vi "HW_Gantner_Get Save T0.vi"(5 "dt":dbl format="%#_13g", 7 "data length":i32, 9 "error in":errorcluster, 10 "StartT0":timestamp, 11 "T0 in":timestamp) -> (1 "error out":errorcluster, 2 "TimeCh data":waveform(dbl), 3 "T0 out":timestamp)   [LabVIEW 2016]
uses:
  Ctrls/Continuous Operations.ctl
  Ctrls/GlobeVaribles.vi
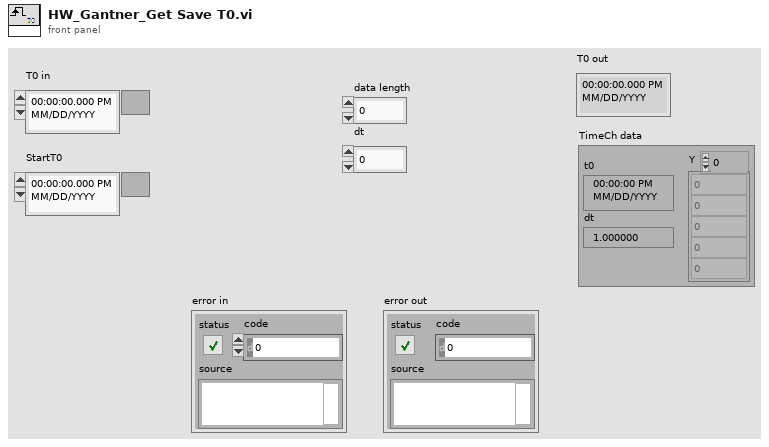
[diagram p1: front panel]
types:
  T1 = typedef "Continuous Operations.ctl" = enum16{"Writting", "Pause", "Stop"}
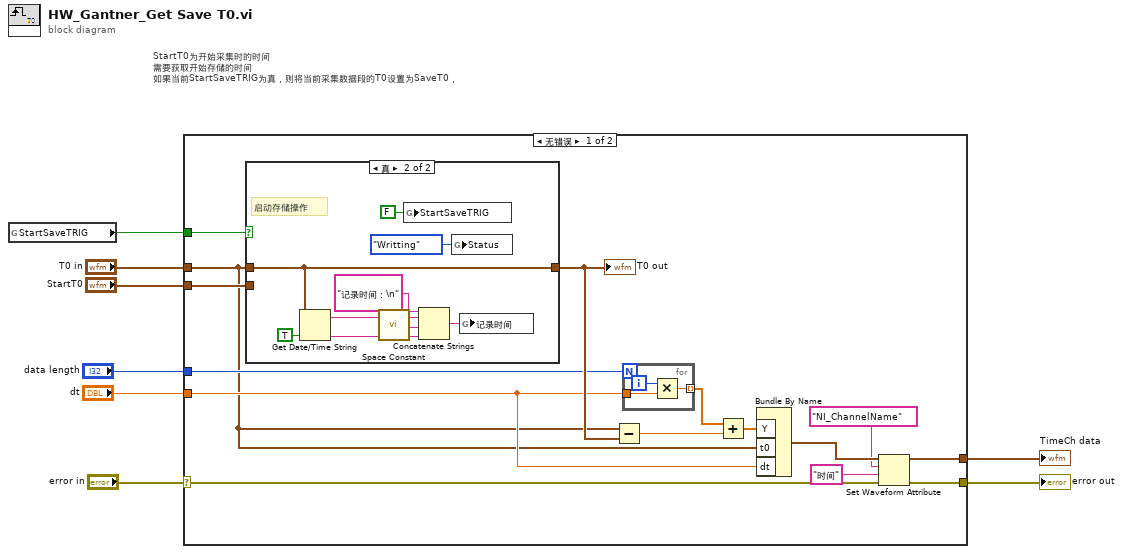
[diagram p0: block diagram]
diagram:
  # "StartT0为开始采集时的时间\n需要获取开始存储的时间\n如果当前StartSaveTRIG为真，则将当前采集数据段的T0设置为SaveT0，"
  n1 = global read "GlobeVaribles.vi" "StartSaveTRIG"() -> (w7:bool)
  n2 = case shown="无错误" "error in" {
    selector: "error in" -> [w12 w37]
    tunnel: "StartT0" -> [w23 _]
    tunnel: w7 -> [w22 _]
    tunnel: "T0 in" -> [w10 _]
    tunnel: "data length" -> [w14 _]
    tunnel: "dt" -> [w13 _]
    tunnel: [w11 w37] -> w2
    tunnel: [w9 _] -> w1
    frame No Error {
      n3 = case shown="真" w22 {
        tunnel: w10 -> [_ w34]
        tunnel: [w27 w34] -> w15
        tunnel: w23 -> [w27 _]
        frame False {
        }
        frame True {
          # "启动存储操作"
          n4 = Get Date/Time String(seconds (now)=w34, want seconds? (F)=TRUE ("需要秒？(F)")) -> (date string=w33:string, time string=w32:string)  [unwired: 1 in]
          n5 = call <vilib>:"Space Constant.vi"() -> ("String"=w29:string)
          n6 = global write "GlobeVaribles.vi" "StartSaveTRIG"(FALSE ("StartSaveTRIG")) -> ()
          n7 = Concatenate Strings("记录时间：\n" ("字符串"), w33, w29, w32) -> (w31:string)
          n8 = global write "GlobeVaribles.vi" "Status"(Continuous_Operations."Writting" ("Status")) -> ()
          n9 = global write "GlobeVaribles.vi" "记录时间"(w31) -> ()
        }
      }
      "T0 out" <- w15
      n10 = Subtract(x=w10, y=w15) -> (x-y=w19:dbl)
      n11 = for {
        N: w14 -> [_]
        tunnel: w13 -> [w25]
        tunnel: [w24] -> w21 mode=indexing
        i -> [w26]
        n12 = Multiply(x=w26, y=w25) -> (x*y=w24:dbl)
      }
      n13 = Add(x=w21, y=w19) -> (x+y=w20:dbl[])
      n14 = Bundle By Name("Y"=w20, "t0"=w10, "dt"=w13) -> (w18:waveform(dbl))  [unwired: 1 in]
      n15 = Set Waveform Attribute(4:w12, 5:"时间" ("名称"), 6:"NI_ChannelName" ("名称"), 7:w18) -> (0:w11:errorcluster, 3:w9:waveform(dbl))  [unwired: 1 out]
    }
    frame Error {
    }
  }
  "error out" <- w2
  "TimeCh data" <- w1
